vi "ListWorkSheetNames.vi"(8 "error in (no error)":errorcluster, 11 "ExcelFile in":refnum<class "PortableExcelFileManipulationOXML.lvclass">) -> (0 "error out":errorcluster, 2 "Array":string[](array[string]), 3 "ExcelFile out":refnum<class "PortableExcelFileManipulationOXML.lvclass">)   [LabVIEW 2019, in "PortableExcelFileManipulationOXML.lvclass"]
doc: "Adds a worksheet to the This excel File by name."
uses:
  PortableExcelFileManipulationOXML.lvclass
  PortableExcelFileManipulationOXML.lvclass/PortableExcelFileManipulationOXML.ctl
  H:/LV projects/ExpressionEvaluator/Excel/ExcelManipulation.dll
  ExcelManipulation.dll
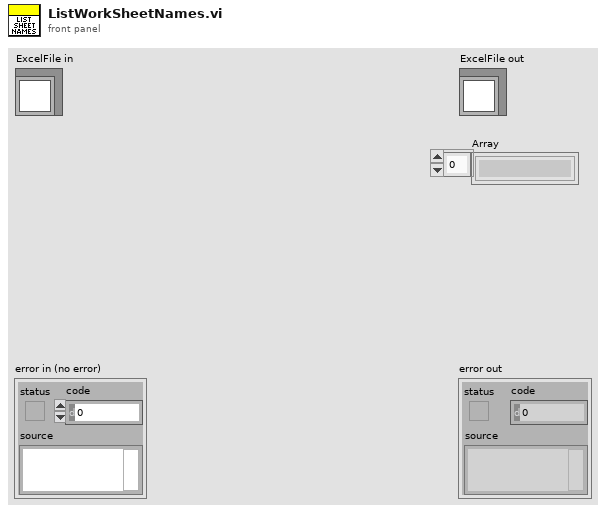
[diagram p1: front panel]
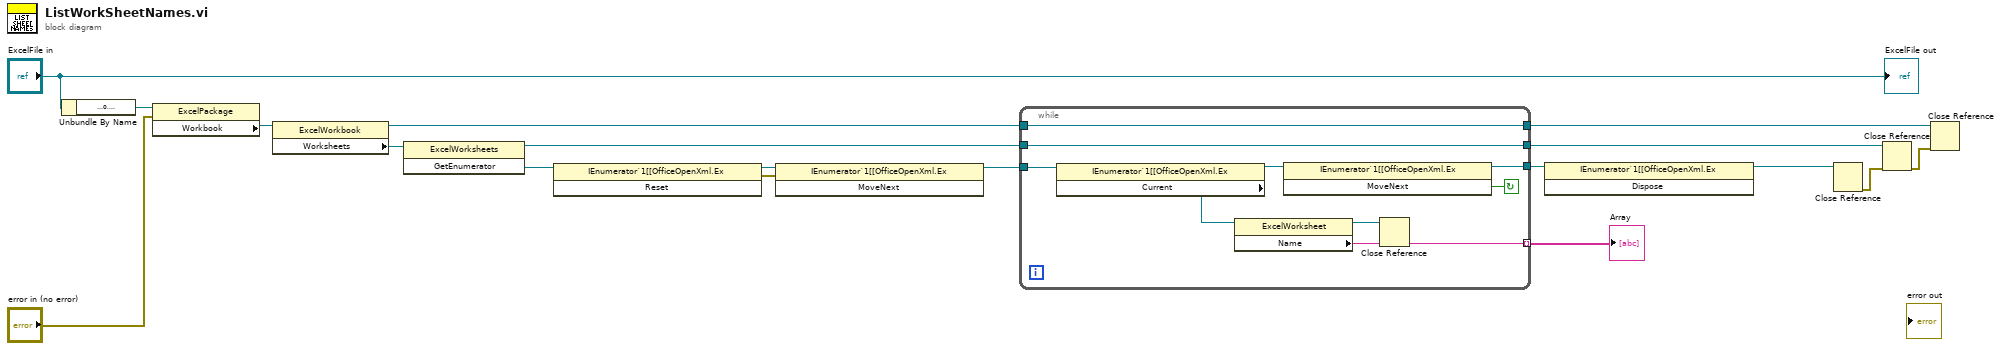
[diagram p0: block diagram]
diagram:
  n1 = Unbundle By Name("ExcelFile in") -> ("ExcelOpen"=w17:refnum<k24>)
  n2 = property class="ExcelPackage"(reference=w17, error in="error in (no error)") -> ("Workbook"=w16:refnum<k24>)  [unwired: 2 out]
  n3 = property class="ExcelWorkbook"(reference=w16) -> (reference out=w2:refnum<k24>, "Worksheets"=w14:refnum<k24>)  [unwired: 1 in, 1 out]
  n4 = invoke class="ExcelWorksheets" method="GetEnumerator"(reference=w14) -> (reference out=w6:refnum<k24>, "GetEnumerator"=w13:refnum<k24>)  [unwired: 2 in, 1 out]
  n5 = invoke class="IEnumerator`1[[OfficeOpenXml.Ex" method="Reset"(reference=w13) -> (reference out=w11:refnum<k24>, error out=w12:errorcluster)  [unwired: 2 in, 1 out]
  n6 = invoke class="IEnumerator`1[[OfficeOpenXml.Ex" method="MoveNext"(reference=w11, error in=w12) -> (reference out=w10:refnum<k24>)  [unwired: 1 in, 2 out]
  n7 = while {
    tunnel: w10 -> [w27]
    tunnel: [w24] -> w9 mode=indexing
    tunnel: [w22] -> w8
    tunnel: w6 -> [w21]
    tunnel: [w21] -> w4
    tunnel: w2 -> [w20]
    tunnel: [w20] -> w1
    stop <- w23 continue-if-true
    n8 = property class="IEnumerator`1[[OfficeOpenXml.Ex"(reference=w27) -> (reference out=w25:refnum<k24>, "Current"=w26:refnum<k24>)  [unwired: 1 in, 1 out]
    n9 = property class="ExcelWorksheet"(reference=w26) -> (reference out=w19:refnum<k24>, "Name"=w24:string)  [unwired: 1 in, 1 out]
    n10 = invoke class="IEnumerator`1[[OfficeOpenXml.Ex" method="MoveNext"(reference=w25) -> (reference out=w22:refnum<k24>, "MoveNext"=w23:bool)  [unwired: 2 in, 1 out]
    n11 = Close Reference(reference=w19) -> ()  [unwired: 1 in, 1 out]
  }
  "Array" <- w9
  n12 = invoke class="IEnumerator`1[[OfficeOpenXml.Ex" method="Dispose"(reference=w8) -> (reference out=w7:refnum<k24>)  [unwired: 2 in, 2 out]
  n13 = Close Reference(reference=w7) -> (error out=w5:errorcluster)  [unwired: 1 in]
  n14 = Close Reference(reference=w4, error in (no error)=w5) -> (error out=w3:errorcluster)
  n15 = Close Reference(reference=w1, error in (no error)=w3) -> ()  [unwired: 1 out]
  "ExcelFile out" <- "ExcelFile in"
